vi "Config GUI - Spamming Has Stopped.vi"(8 "Error In":errorcluster, 11 "GUI refs":T1) -> (0 "Error Out":errorcluster)   [LabVIEW 2016, in "Anti-Spam Tester (AST).lvlib"]
doc: "The spamming is stopped. Configure the GUI in such a way that the user can configure a new series of spamming (can change the values of spamming inputs)."
uses:
  Anti-Spam Tester (AST).lvlib
  Spam Mode (enum).ctl
  Spam Frequency (enum).ctl
  Spam Error Message Type (enum).ctl
  GUI refs - Input (cluster).ctl
  GUI refs - Buttons (cluster).ctl
  GUI refs (cluster).ctl
panel:
  # "Input\nInputs to the VI"
  # "Development\nControls or indicators that are useful for development or testing, but which are not outputs of the VI."
  # "Output\nOutputs of the VI"
  # "Description\n\nBlank VI with error handling case. \n\nSummarize the use of this VI in this space."
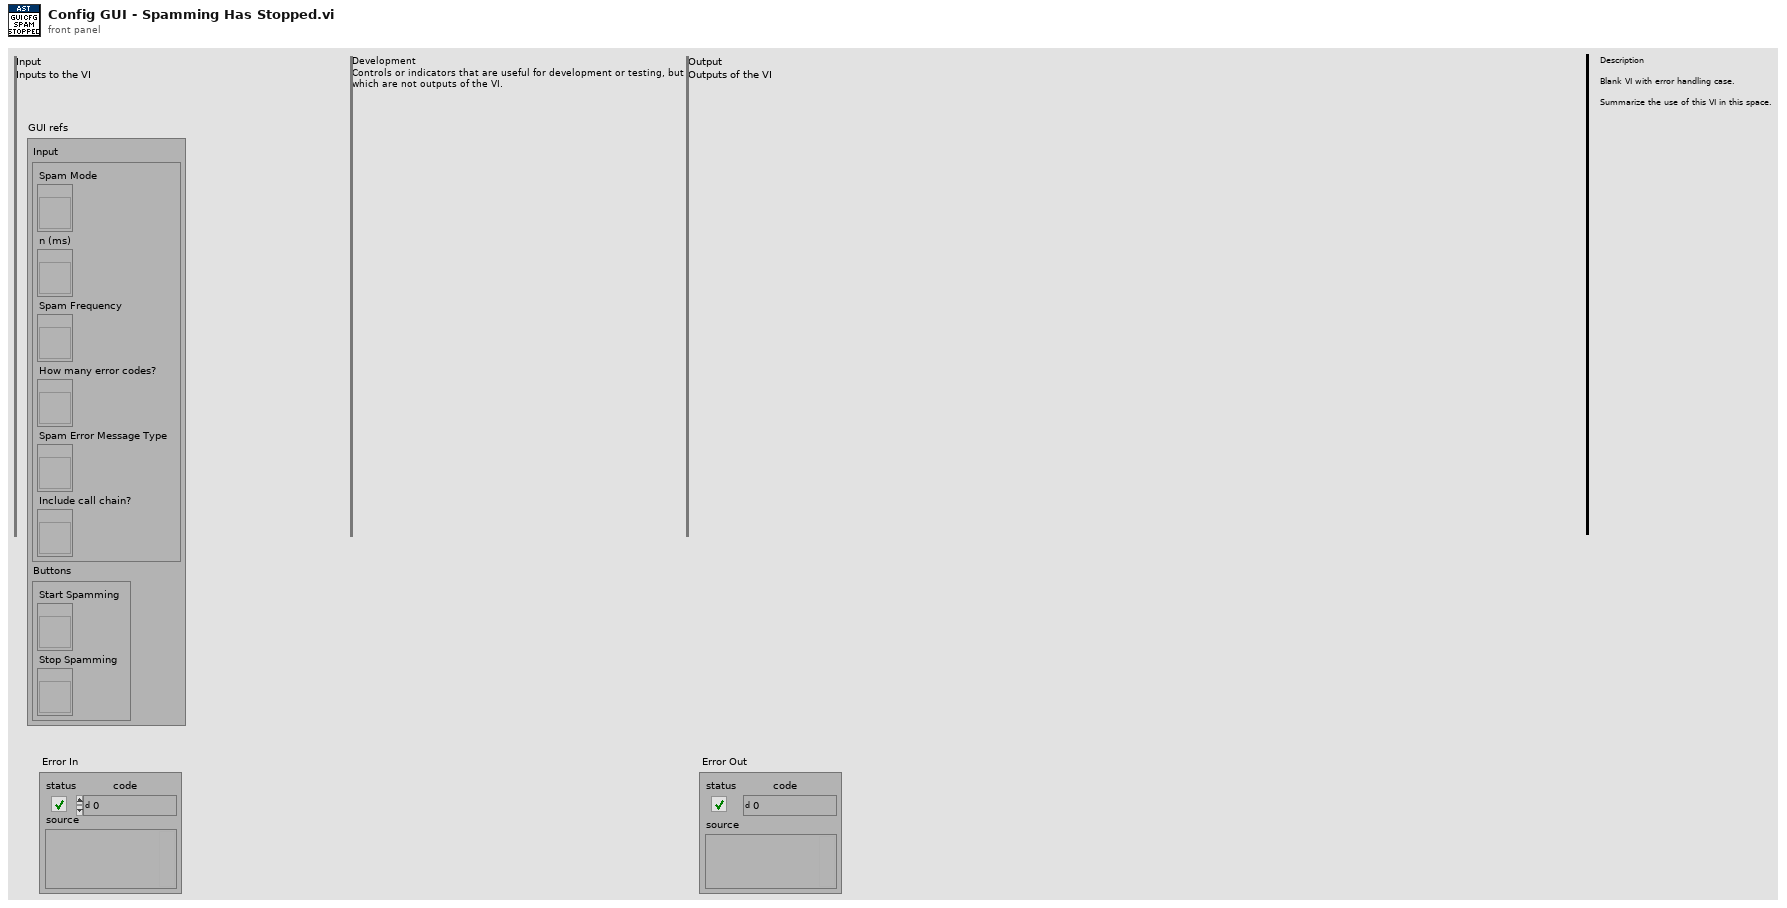
[diagram p1: front panel]
types:
  T1 = typedef "Anti-Spam Tester (AST).lvlib/GUI refs (cluster).ctl" = cluster{"Input":T2, "Buttons":T3}
  T2 = typedef "Anti-Spam Tester (AST).lvlib/GUI refs - Input (cluster).ctl" = cluster{"Spam Mode":refnum<vi>, "n (ms)":refnum<vi>, "Spam Frequency":refnum<vi>, "How many error codes?":refnum<vi>, "Spam Error Message Type":refnum<vi>, "Include call chain?":refnum<vi>}
  T3 = typedef "Anti-Spam Tester (AST).lvlib/GUI refs - Buttons (cluster).ctl" = cluster{"Start Spamming":refnum<vi>, "Stop Spamming":refnum<vi>}
  T4 = enum8{"Enabled", "Disabled", "Disabled and Grayed Out"}
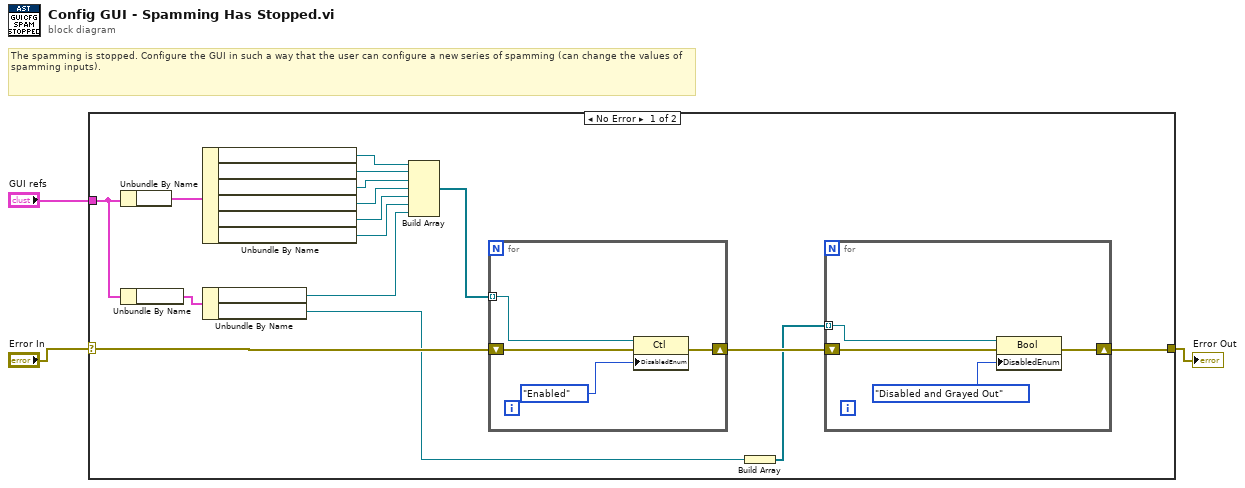
[diagram p0: block diagram]
diagram:
  # "The spamming is stopped. Configure the GUI in such a way that the user can configure a new series of spamming (can change the values of spamming inputs)."
  n1 = case shown="No Error" "Error In" {
    selector: "Error In" -> [w19 w28]
    tunnel: [w16 w28] -> w2
    tunnel: "GUI refs" -> [w8 _]
    frame No Error {
      n2 = Unbundle By Name(w8) -> (w18:T2)
      n3 = Unbundle By Name(w8) -> (w7:T3)
      n4 = Unbundle By Name(w18) -> (w15:refnum<vi>, w14:refnum<vi>, w13:refnum<vi>, w12:refnum<vi>, w11:refnum<vi>, w10:refnum<vi>)
      n5 = Unbundle By Name(w7) -> (w6:refnum<vi>, w5:refnum<vi>)
      n6 = Build Array(w15, w14, w13, w12, w11, w10, w6) -> (w9:refnum<vi>[])
      n7 = for {
        shift-right: [w25] -> w17
        shift-left: w19 -> [w27]
        tunnel: w9 -> [w24] mode=indexing
        n8 = property class="Ctl"(reference=w24, error in=w27, "DisabledEnum"=T4."Enabled" ("Disabled")) -> (error out=w25:errorcluster)  [unwired: 1 out]
      }
      n9 = Build Array(w5) -> (w4:refnum<vi>[])
      n10 = for {
        shift-right: [w21] -> w16
        shift-left: w17 -> [w22]
        tunnel: w4 -> [w20] mode=indexing
        n11 = property class="Bool"(reference=w20, error in=w22, "DisabledEnum"=T4."Disabled and Grayed Out" ("Disabled")) -> (error out=w21:errorcluster)  [unwired: 1 out]
      }
    }
    frame Error {
    }
  }
  "Error Out" <- w2
